vi "Analysis.Main.vi"(6 "Refs":T1, 8 "error in (no error)":errorcluster, 9 "Headers":string[](array[string]), 10 "Data Path":path, 11 "Result Directory":path) -> (0 "error out":errorcluster, 3 "Overall Result":bool)   [LabVIEW 2014, in "NIAnalysis.lvlib"]
uses:
  NIAnalysis.lvlib
  Types/AnalysisGUI.Refs.ctl
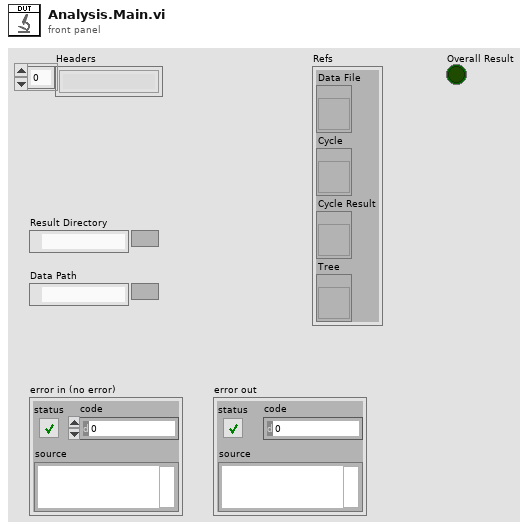
[diagram p1: front panel]
types:
  T1 = typedef "NIAnalysis.lvlib/AnalysisGUI.Refs.ctl" = cluster{"Data File":refnum<vi>, "Cycle":refnum<vi>, "Cycle Result":refnum<vi>, "Tree":refnum<vi>}
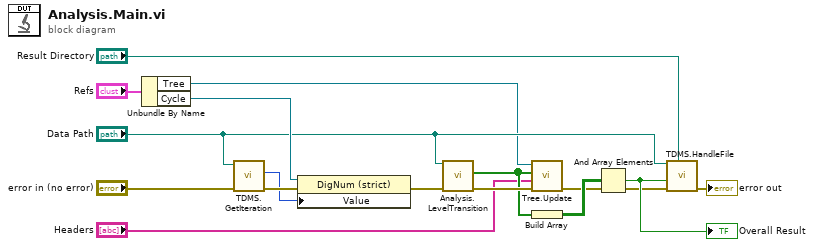
[diagram p0: block diagram]
diagram:
  n1 = Unbundle By Name("Refs") -> ("Tree"=w6:refnum<vi>, "Cycle"=w13:refnum<vi>)
  n2 = call "TDMS.GetIteration.vi"("error in (no error)"="error in (no error)", "Data"="Data Path") -> ("error out"=w11:errorcluster, "Iteration"=w8:i32)  [unwired: 8 in]
  n3 = property class="DigNum (strict)"(reference=w13, error in=w11, "Value"=w8) -> (error out=w4:errorcluster)  [unwired: 1 out]
  n4 = call "Analysis.LevelTransition.vi"("error in"=w4, "Data"="Data Path") -> ("error out"=w12:errorcluster, "Result"=w10:bool[])  [unwired: 7 in, 1 out]
  n5 = call "Tree.Update.vi"("error in (no error)"=w12, "Analysis Tags"="Headers", "Result"=w10, "TreeControl in"=w6) -> ("error out"=w3:errorcluster)  [unwired: 6 in, 1 out]
  n6 = Build Array(w10) -> (w9:bool[][])
  n7 = And Array Elements(Boolean array=w9) -> (logical AND=w15:bool)
  "Overall Result" <- w15
  n8 = call "TDMS.HandleFile.vi"("Result Directory"="Result Directory", "error out"=w3, "Delete"=w15, "Data"="Data Path") -> ("error out"=→"error out":errorcluster)  [unwired: 6 in, 1 out]
